vi "cube vision.vi"(11 "Image":T1=refnum) -> (3 "angle":dbl=-4.632444083491556)   [LabVIEW 2017]
uses:
  <vilib>/vision/Image Controls.llb/IMAQ Image.ctl
panel:
  out "Color":T1(plugin-control)
  out "Binary Image":T1(plugin-control)
  in  "Sat Range":cluster{u8, u8}(slide)={255, 210} scale=0.0..255.0
  in  "Hue Range":cluster{u8, u8}(slide)={67, 19} scale=0.0..255.0
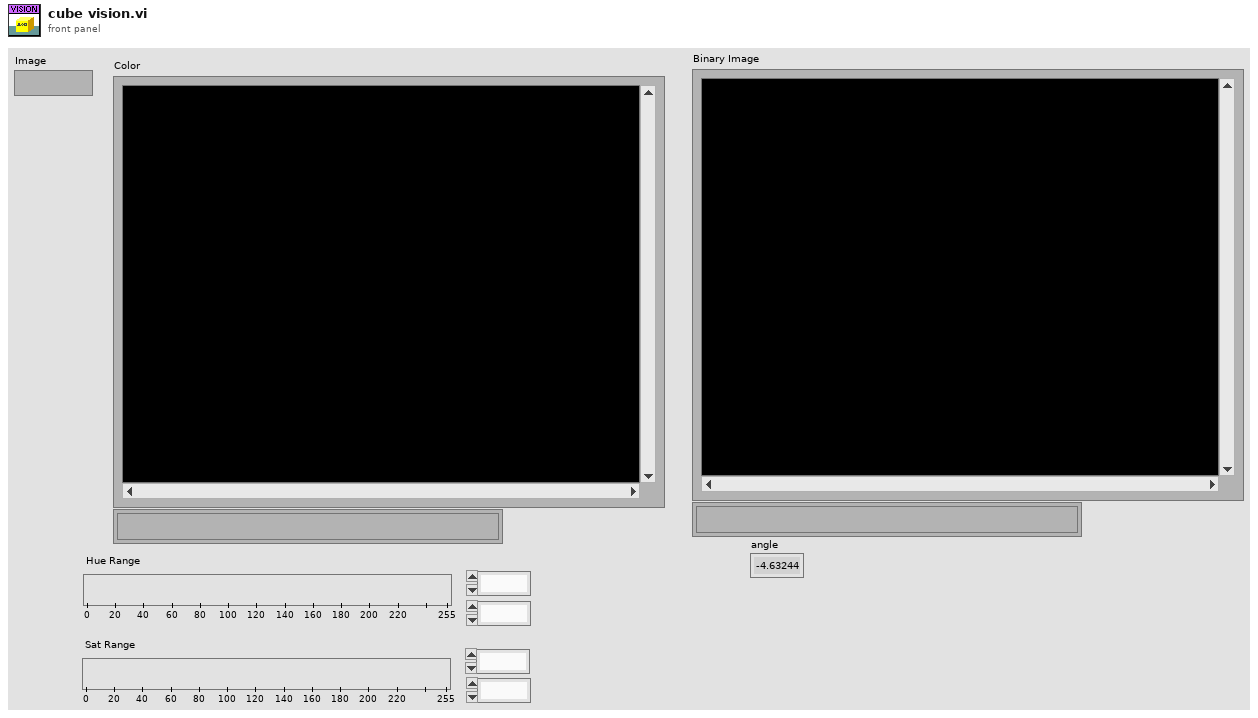
[diagram p1: front panel]
types:
  T1 = typedef "IMAQ Image.ctl" = refnum<image>
  T2 = typedef "Image Type" = u32
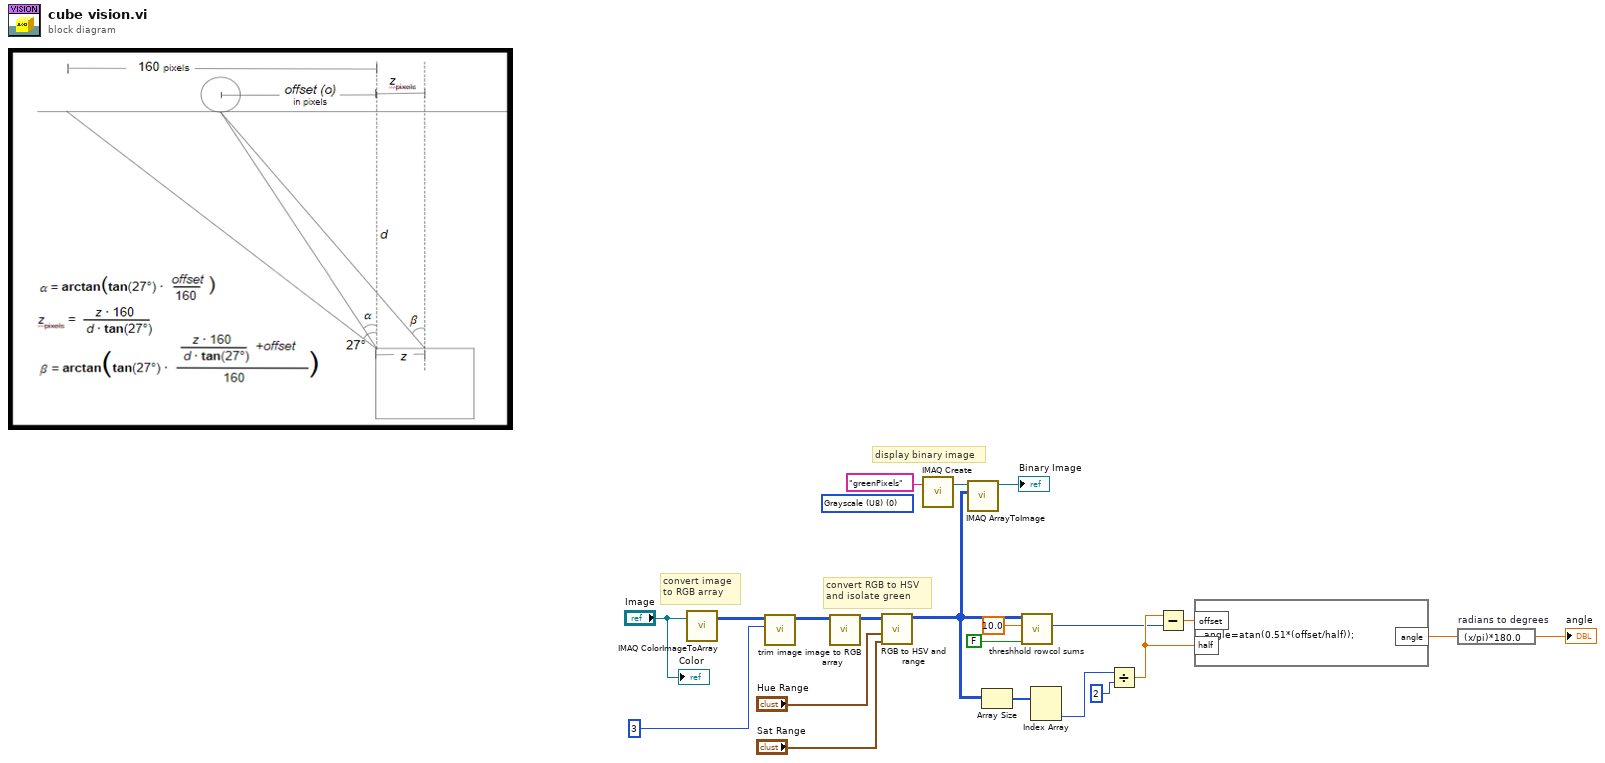
[diagram p0: block diagram]
diagram:
  (unwired) T2 0 items=["Grayscale (U8)", "Grayscale (I16)", "Grayscale (SGL)", "Complex (CSG)", "RGB (U32)", "HSL (U32)", "RGB (U64)", "Grayscale (U16)"] ("Image Type")
  # "display binary image"
  # "convert image\nto RGB array"
  # "convert RGB to HSV\nand isolate green"
  n1 = call "IMAQ ColorImageToArray"("Image"="Image") -> ("Image Pixels (U32)"=w3:u32[][])  [unwired: 3 in, 2 out]
  n2 = call "trim image.vi"("scale"=3, "Image Pixels (U32)"=w3) -> ("Trimmed Image Pixels (U32)"=w2:u32[][])  [unwired: 9 in]
  n3 = call "image to RGB array.vi"("Image Pixels (U32)"=w2) -> ("Image Pixels (U8)"=w21:u8[][][])  [unwired: 10 in]
  n4 = call "RGB to HSV and range.vi"("Image Pixels (RGB)"=w21, "Hue Range"="Hue Range", "Sat Range"="Sat Range") -> ("Threshholded Pixels"=w12:u8[][])  [unwired: 7 in]
  n5 = call "IMAQ Create"("Image Name"="greenPixels") -> ("New Image"=w17:T1)  [unwired: 4 in, 1 out]
  n6 = call "IMAQ ArrayToImage"("Image Pixels (U8)"=w12, "Image"=w17) -> ("Image Out"=→"Binary Image":T1)  [unwired: 8 in, 1 out]
  n7 = Array Size(array=w12) -> (size(s)=w13:i32[])
  n8 = call "threshhold rowcol sums.vi"("Row(T)/Col(F)"=FALSE, "Threshold"=10.0, "Pixels"=w12) -> ("middle row/col"=w5:i32)  [unwired: 6 in, 2 out]
  n9 = Index Array(array=w13) -> (element #2=w11:i32)  [unwired: 2 in, 1 out]
  n10 = Divide(x=w11, y=2) -> (x/y=w6:dbl)
  n11 = Subtract(x=w6, y=w5) -> (x-y=w7:dbl)
  n12 = formula code="angle=atan(0.51*(offset/half));"("offset"=w7, "half"=w6) -> ("angle"=w9:dbl)
  n13 = expression code="(x/pi)*180.0" "radians to degrees"(w9) -> (→"angle":dbl)
  "Color" <- "Image"
